vi "process_storage.vi"() -> ()   [LabVIEW 2011, in "Fiberscope_library.lvlib"]
uses:
  Fiberscope_library.lvlib
  typedefs/element_images_cluster.ctl
  typedefs/control_process_state_cluster.ctl
  typedefs/control_process_state_enum.ctl
  typedefs/feedback_to_watchdog.ctl
  typedefs/feedback_from_process_enum.ctl
  typedefs/all_scan_parameters_cluster.ctl
  typedefs/fiber_parameters_cluster.ctl
  typedefs/spiral_parameters_cluster.ctl
  typedefs/run_parameters_cluster.ctl
  typedefs/run_mode_enum.ctl
  typedefs/acquisition_parameters_cluster.ctl
  typedefs/image_size_I32.ctl
  typedefs/smooth_coeffs_cluster.ctl
  typedefs/storage_parameters_cluster.ctl
panel:
  out "Local exit":bool
  out "Last saved image":string
  out "error out":errorcluster
  in  "error in":errorcluster
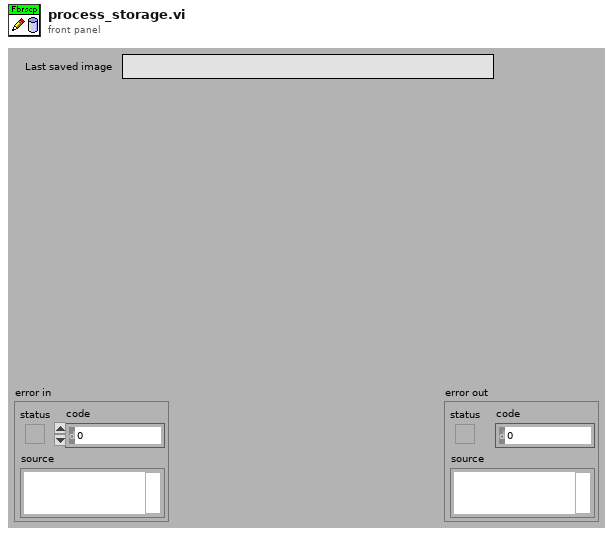
[diagram p1: front panel]
types:
  T1 = typedef "Fiberscope_library.lvlib/feedback_to_watchdog.ctl" = cluster{"Feedback_from_process_enum":T2, "Process_name":string}
  T2 = typedef "Fiberscope_library.lvlib/feedback_from_process_enum.ctl" = enum16{"Has_initialised", "Changed_parameters", "Has_started", "Has_stopped", "Has_quitted", "Is_running", "Has_finished", "Custom"}
  T3 = typedef "Fiberscope_library.lvlib/control_process_state_cluster.ctl" = cluster{"Control_process_state_enum":T4, "variant":variant}
  T4 = typedef "Fiberscope_library.lvlib/control_process_state_enum.ctl" = enum16{"Init", "Quit", "Start", "Stop", "Change_parameters", "Running", "Finish", "Custom"}
  T5 = typedef "Fiberscope_library.lvlib/element_images_cluster.ctl" = cluster{"Images_array":dbl[][][], "#channels":i32, "Last element?":bool}
  T6 = typedef "Fiberscope_library.lvlib/all_scan_parameters_cluster.ctl" = cluster{"Fiber parameters":T7, "Spiral parameters":T8, "Run parameters":T9, "Acquisition parameters":T11, "Fiber parameters pixel_mapper":T7, "Smooth_coeffs_cluster":T13, "Storage parameters":T14}
  T7 = typedef "Fiberscope_library.lvlib/fiber_parameters_cluster.ctl" = cluster{"Frequency":dbl, "Amplitude X":dbl, "Amplitude Y":dbl, "Initial Amplitude X":dbl, "Initial Amplitude Y":dbl, "Phase":dbl}
  T8 = typedef "Fiberscope_library.lvlib/spiral_parameters_cluster.ctl" = cluster{"Imaging periods":dbl, "Settling periods":dbl, "Resting periods":dbl}
  T9 = typedef "Fiberscope_library.lvlib/run_parameters_cluster.ctl" = cluster{"Run mode":T10, "Averages per frame":u8, "No. of frames":u32}
  T10 = typedef "Fiberscope_library.lvlib/run_mode_enum.ctl" = enum16{"Continuous", "Single frame", "No. of frames"}
  T11 = typedef "Fiberscope_library.lvlib/acquisition_parameters_cluster.ctl" = cluster{"Cycles per pixel":u32, "Image size":T12}
  T12 = typedef "Fiberscope_library.lvlib/image_size_I32.ctl" = i32
  T13 = typedef "Fiberscope_library.lvlib/smooth_coeffs_cluster.ctl" = cluster{"Coeff 1":dbl, "Coeff 2":dbl}
  T14 = typedef "Fiberscope_library.lvlib/storage_parameters_cluster.ctl" = cluster{"Autosave":bool, "Path":path}
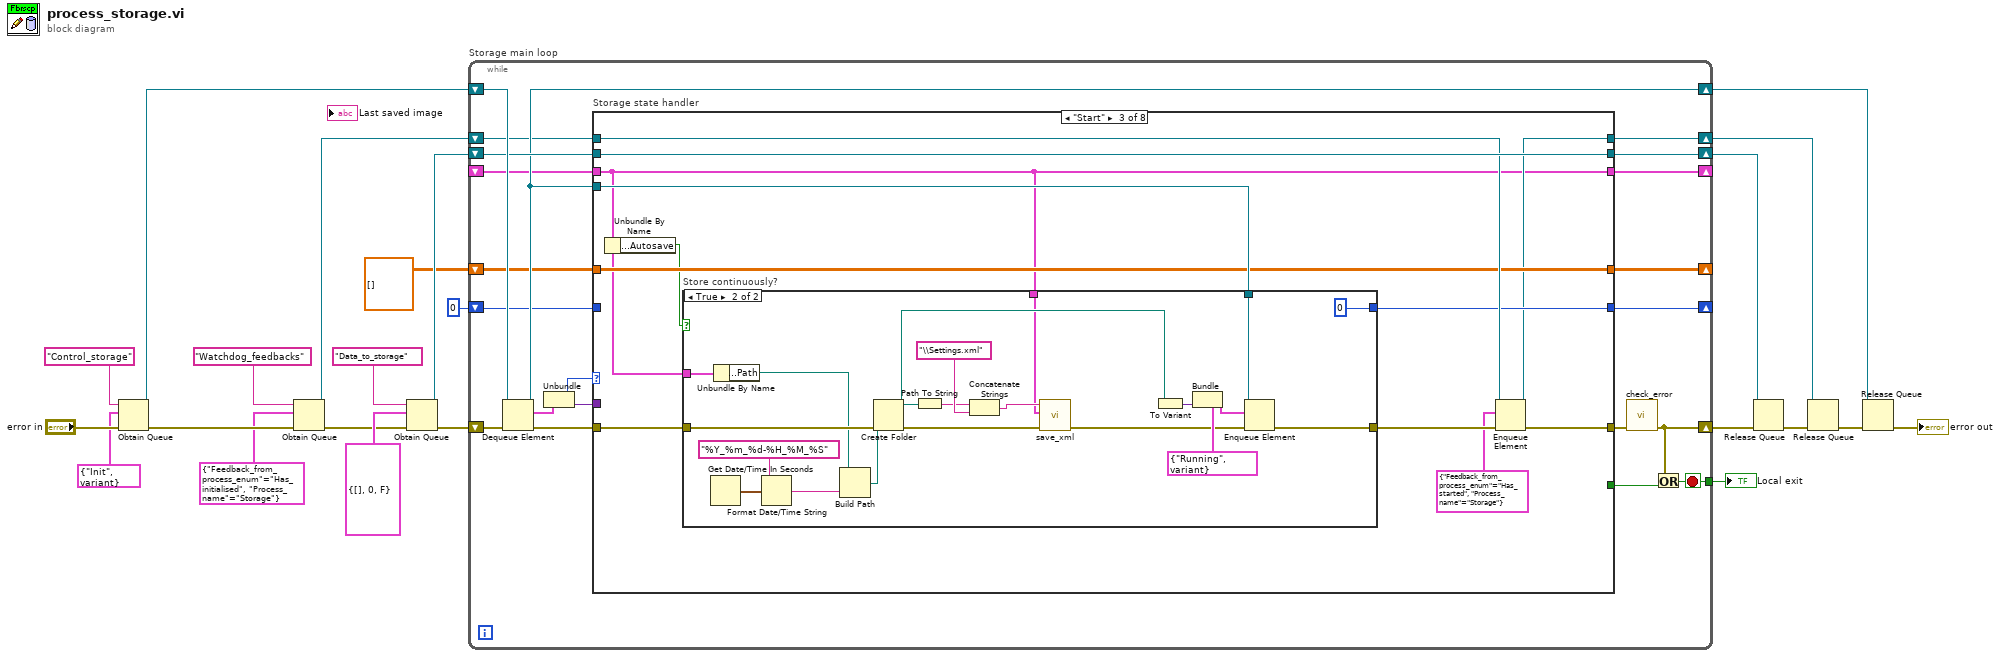
[diagram p0: block diagram]
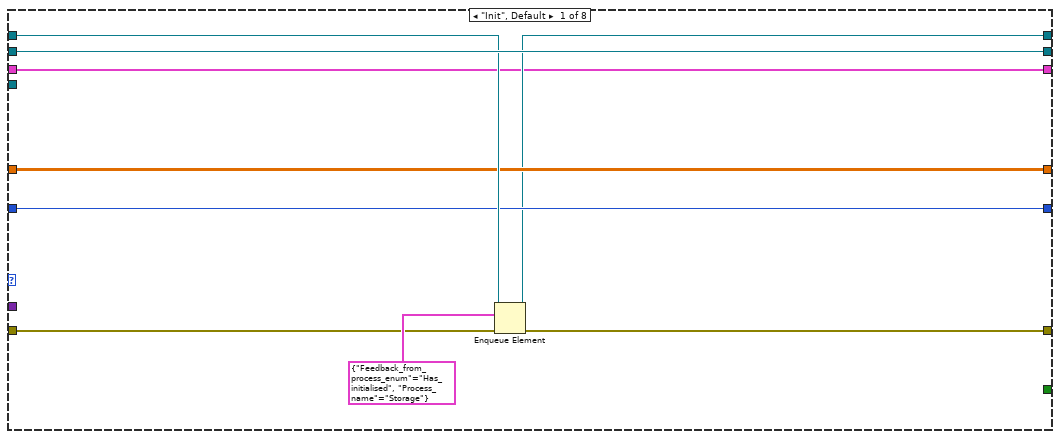
[diagram p2: hidden frame]
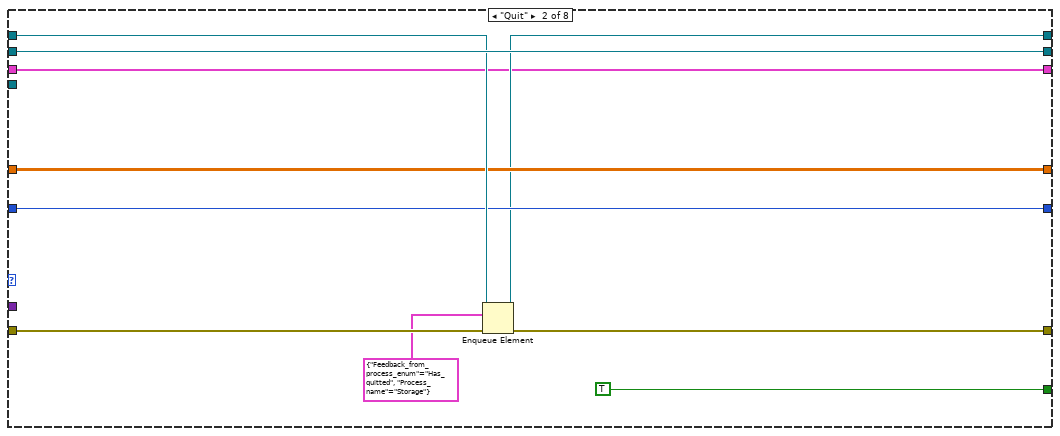
[diagram p3: hidden frame]
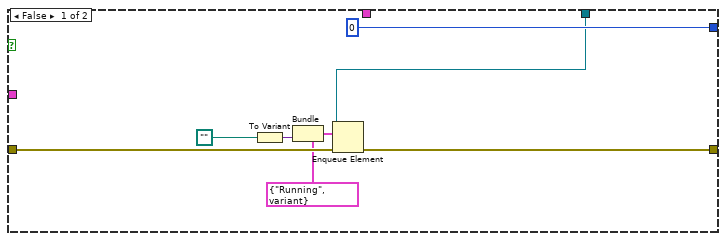
[diagram p4: hidden frame]
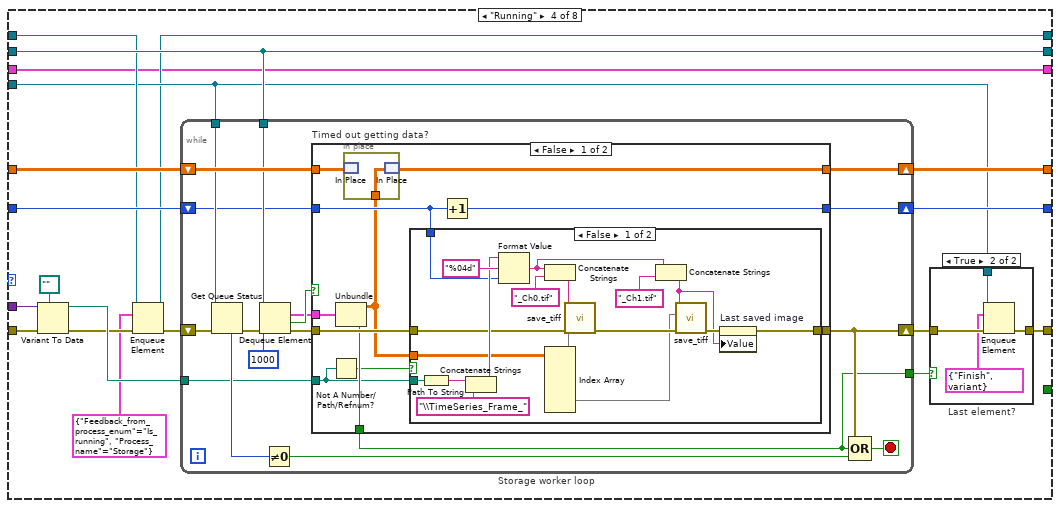
[diagram p5: hidden frame]
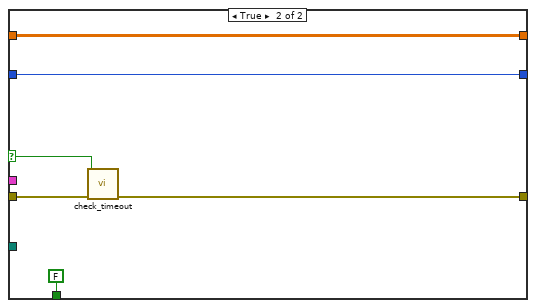
[diagram p8: hidden frame]
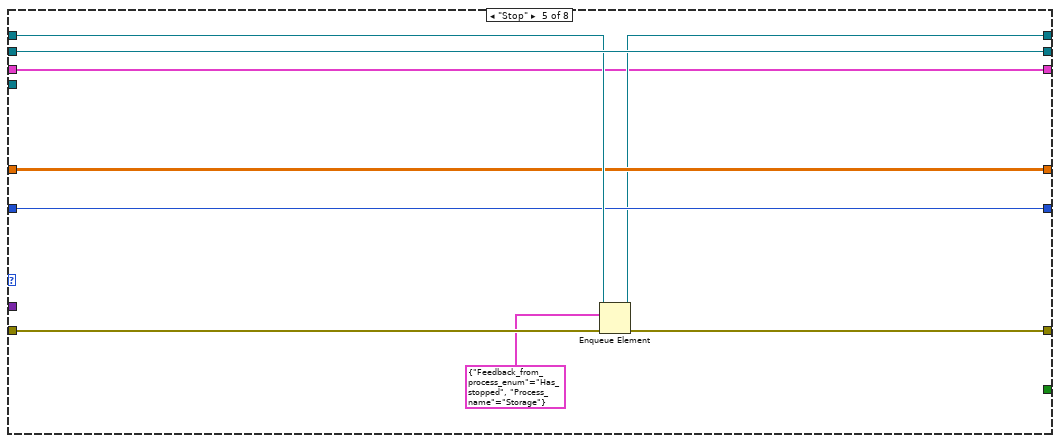
[diagram p9: hidden frame]
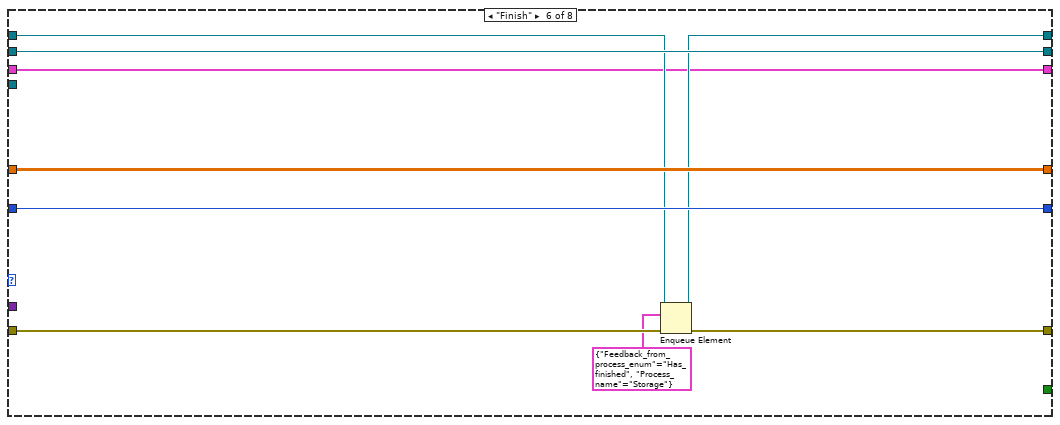
[diagram p10: hidden frame]
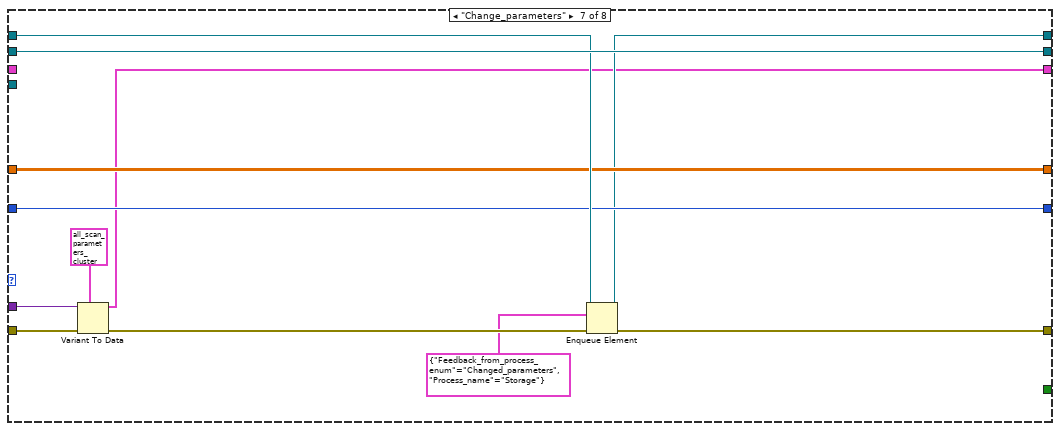
[diagram p11: hidden frame]
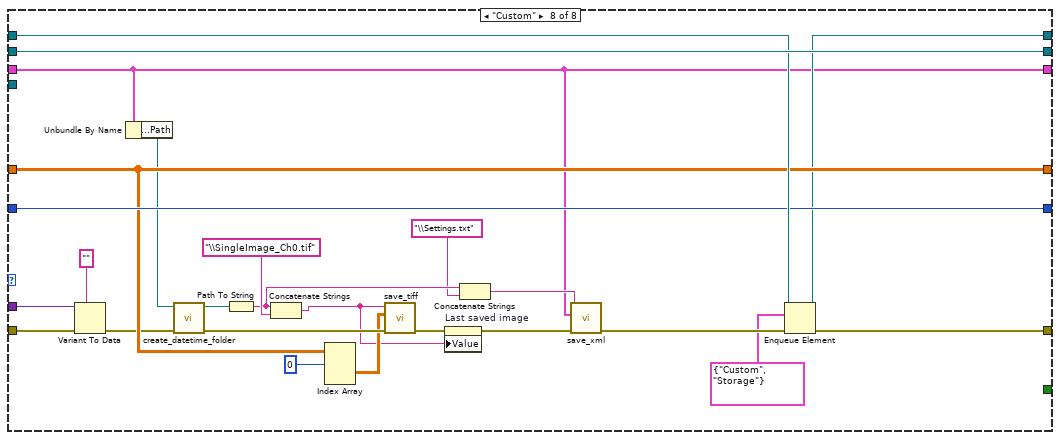
[diagram p12: hidden frame]
diagram:
  n1 = Obtain Queue(name (unnamed)="Control_storage", element data type=T3 {"Control_process_state_enum"=enum."Init", "variant"=variant} ("Control_process_state_cluster"), error in (no error)="error in") -> (queue out=w7:refnum<queue>, error out=w6:errorcluster)  [unwired: 2 in, 1 out]
  n2 = Obtain Queue(name (unnamed)="Watchdog_feedbacks", element data type=T1 {"Feedback_from_process_enum"=enum."Has_initialised", "Process_name"="Storage"}, error in (no error)=w6) -> (queue out=w12:refnum<queue>, error out=w14:errorcluster)  [unwired: 2 in, 1 out]
  n3 = Obtain Queue(name (unnamed)="Data_to_storage", element data type=T5 {"Images_array"=[], "#channels"=0, "Last element?"=FALSE}, error in (no error)=w14) -> (queue out=w19:refnum<queue>, error out=w20:errorcluster)  [unwired: 2 in, 1 out]
  n4 = while "Storage main loop" {
    shift-right: [w27] -> w17
    shift-left: w20 -> [w44]
    shift-right: [w35] -> w15
    shift-left: w7 -> [w43]
    shift-right: [w37] -> w16
    shift-left: w19 -> [w38]
    shift-right: [w26] -> w9
    shift-left: w12 -> [w33]
    shift-right: [w32] -> _
    shift-left: dbl[][][] [] ("Images_array") -> [w31]
    tunnel: [w30] -> w8
    shift-right: [w29] -> _
    shift-left: 0 -> [w28]
    shift-right: [w25] -> _
    shift-left: _ -> [w24]
    stop <- w30 stop-if-true
    n5 = Dequeue Element(queue=w43, error in (no error)=w44) -> (queue out=w35:refnum<queue>, element=w41:T3, error out=w42:errorcluster)  [unwired: 1 in, 1 out]
    n6 = Unbundle(w41) -> ("Control_process_state_enum"=w40:T4, "variant"=w34:variant)
    n7 = case "Storage state handler" shown="\"Start\"" w40 {
      tunnel: w42 -> [w45 w61 w72 w120 w190 w197 w211 w225]
      tunnel: [w52 w60 w68 w109 w189 w196 w208 w236] -> w36
      tunnel: [_ TRUE _ _ _ _ _ _] -> w39
      tunnel: w38 -> [w53 w62 w75 w115 w191 w200 w212 w237]
      tunnel: [w53 w62 w75 w115 w191 w200 w212 w237] -> w37
      tunnel: w35 -> [_ _ w73 w108 _ _ _ _]
      tunnel: w34 -> [_ _ _ w119 _ _ w210 w223]
      tunnel: w33 -> [w51 w59 w74 w111 w188 w195 w207 w235]
      tunnel: [w50 w58 w71 w122 w187 w199 w206 w228] -> w32
      tunnel: w31 -> [w50 w58 w71 w121 w187 w199 w206 w228]
      tunnel: [w49 w57 w70 w116 w186 w198 w205 w230] -> w29
      tunnel: w28 -> [w49 w57 _ w117 w186 w198 w205 w230]
      tunnel: [w48 w56 w67 w106 w185 w194 w204 w217] -> w26
      tunnel: [w46 w54 w64 w104 w183 w192 w202 w213] -> w25
      tunnel: w24 -> [w46 w54 w64 w104 w183 w192 _ w213]
      frame "Init", Default {
        n8 = Enqueue Element(queue=w51, element=T1 {"Feedback_from_process_enum"=enum."Has_initialised", "Process_name"="Storage"}, error in (no error)=w45) -> (queue out=w48:refnum<queue>, error out=w52:errorcluster)  [unwired: 1 in, 1 out]
      }
      frame "Quit" {
        n9 = Enqueue Element(queue=w59, element=T1 {"Feedback_from_process_enum"=enum."Has_quitted", "Process_name"="Storage"}, error in (no error)=w61) -> (queue out=w56:refnum<queue>, error out=w60:errorcluster)  [unwired: 1 in, 1 out]
      }
      frame "Start" {
        n10 = Unbundle By Name(w64) -> ("Storage parameters.Autosave"=w65:bool)
        n11 = case "Store continuously?" shown="True" w65 {
          tunnel: w73 -> [w80 w103]
          tunnel: w72 -> [w82 w98]
          tunnel: [0 0] -> w70
          tunnel: [w81 w96] -> w69
          tunnel: w64 -> [_ w84]
          tunnel: w64 -> [_ w86]
          frame False {
            n12 = To Variant(anything=path "") -> (Variant=w77:variant)
            n13 = Bundle(cluster=T3 {"Control_process_state_enum"=enum."Running", "variant"=variant} ("Control_process_state_cluster"), "variant"=w77) -> (w78:T3)  [unwired: 1 in]
            n14 = Enqueue Element(queue=w80, element=w78, error in (no error)=w82) -> (error out=w81:errorcluster)  [unwired: 1 in, 2 out]
          }
          frame True {
            n15 = Get Date/Time In Seconds() -> (seconds since 1Jan1904=w102:timestamp)
            n16 = Unbundle By Name(w86) -> ("Storage parameters.Path"=w85:path)
            n17 = Format Date/Time String(time format string (%c)="%Y_%m_%d-%H_%M_%S", seconds (now)=w102) -> (date/time string=w101:string)  [unwired: 1 in]
            n18 = Build Path(base path=w85, name or relative path=w101) -> (appended path=w99:path)
            n19 = Create Folder(path (use dialog)=w99, error in=w98) -> (created path=w91:path, error out=w88:errorcluster)  [unwired: 1 in, 1 out]
            n20 = Path To String(path=w91) -> (string=w90:string)
            n21 = Concatenate Strings(w90, "\\Settings.xml" ("string")) -> (w89:string)
            n22 = call "save_xml.vi"("error in"=w88, "All scan parameters"=w84, "Path"=w89) -> ("error out"=w87:errorcluster)  [unwired: 8 in]
            n23 = To Variant(anything=w91) -> (Variant=w95:variant)
            n24 = Bundle(cluster=T3 {"Control_process_state_enum"=enum."Running", "variant"=variant} ("Control_process_state_cluster"), "variant"=w95) -> (w94:T3)  [unwired: 1 in]
            n25 = Enqueue Element(queue=w103, element=w94, error in (no error)=w87) -> (error out=w96:errorcluster)  [unwired: 1 in, 2 out]
          }
        }
        n26 = Enqueue Element(queue=w74, element=T1 {"Feedback_from_process_enum"=enum."Has_started", "Process_name"="Storage"}, error in (no error)=w69) -> (queue out=w67:refnum<queue>, error out=w68:errorcluster)  [unwired: 1 in, 1 out]
      }
      frame "Running" {
        n27 = Variant To Data(error in=w120, type=path "" ("Path"), Variant=w119) -> (data=w114:path, error out=w113:errorcluster)
        n28 = Enqueue Element(queue=w111, element=T1 {"Feedback_from_process_enum"=enum."Is_running", "Process_name"="Storage"}, error in (no error)=w113) -> (queue out=w106:refnum<queue>, error out=w112:errorcluster)  [unwired: 1 in, 1 out]
        n29 = while "Storage worker loop" {
          shift-right: [w129] -> w110
          shift-left: w112 -> [w145]
          shift-right: [w136] -> w122
          shift-left: w121 -> [w135]
          shift-right: [w130] -> w116
          shift-left: w117 -> [w131]
          tunnel: w108 -> [w134]
          tunnel: w115 -> [w133]
          tunnel: w114 -> [w132]
          tunnel: [w128] -> w107
          stop <- w142 stop-if-true
          n30 = Get Queue Status(queue=w134, error in (no error)=w145) -> (error out=w144:errorcluster, # elements in queue=w143:i32)  [unwired: 1 in, 6 out]
          n31 = Dequeue Element(queue=w133, timeout in ms (-1)=1000, error in (no error)=w144) -> (element=w137:T5, timed out?=w138:bool, error out=w139:errorcluster)  [unwired: 1 out]
          n32 = Not Equal To 0?(x=w143) -> (x != 0?=w141:bool)
          n33 = case "Timed out getting data?" shown="False" w138 {
            selector: w138 -> [_ w180]
            tunnel: w139 -> [w154 w182]
            tunnel: [w153 w181] -> w129
            tunnel: w137 -> [w152 _]
            tunnel: [w146 w179] -> w136
            tunnel: w135 -> [w148 w179]
            tunnel: w132 -> [w150 _]
            tunnel: w131 -> [w156 w178]
            tunnel: [w155 w178] -> w130
            tunnel: [w151 FALSE ("Last element?")] -> w128
            frame False {
              n34 = Not A Number/Path/Refnum?(number/path/refnum=w150) -> (NaN/Path/Refnum?=w149:bool)
              n35 = Unbundle(w152) -> ("Images_array"=w147:dbl[][][], "Last element?"=w151:bool)  [unwired: 1 out]
              n36 = in-place {
                in-place-border: w147 -> [w157]
                n37 = in-place-match #1(w148) -> ()  [unwired: 1 out]
                n38 = in-place-match #1(w157) -> (w146:dbl[][][])
              }
              n39 = case shown="False" w149 {
                tunnel: w150 -> [w173 _]
                tunnel: w156 -> [w169 _]
                tunnel: w154 -> [w168 w176]
                tunnel: [w166 w176] -> w153
                tunnel: w147 -> [w164 _]
                frame False {
                  n40 = Path To String(path=w173) -> (string=w175:string)
                  n41 = Concatenate Strings(w175, "\\TimeSeries_Frame_" ("string")) -> (w171:string)
                  n42 = Format Value(string ("")=w171, format string="%04d", value (0)=w169) -> (output string=w161:string)
                  n43 = Concatenate Strings(w161, "_Ch0.tif" ("string")) -> (w165:string)
                  n44 = Index Array(array=w164) -> (element #1=w167:dbl[][], element #2=w159:dbl[][])  [unwired: 6 in]
                  n45 = call "save_tiff.vi"("error in (no error)"=w168, "Data"=w167, "Path"=w165) -> ("error out"=w163:errorcluster)  [unwired: 8 in]
                  n46 = Concatenate Strings(w161, "_Ch1.tif" ("string")) -> (w158:string)
                  n47 = call "save_tiff.vi"("error in (no error)"=w163, "Data"=w159, "Path"=w158) -> ("error out"=w162:errorcluster)  [unwired: 8 in]
                  n48 = property on="Last saved image" class="Str"(error in=w162, "Value"=w158) -> (error out=w166:errorcluster)  [unwired: 1 in, 1 out]
                }
                frame True {
                  # "No valid path provided\n-> do not store continuously!"
                }
              }
              n49 = Increment(x=w156) -> (x+1=w155:i32)
            }
            frame True {
              n50 = call "check_timeout.vi"("error in"=w182, "Timeout?"=w180) -> ("error out"=w181:errorcluster)  [unwired: 9 in]
            }
          }
          n51 = Compound Arithmetic op=OR(w129, w128, w141) -> (w142:bool)
        }
        n52 = case "Last element?" shown="True" w107 {
          tunnel: w110 -> [w123 w127]
          tunnel: [w123 w126] -> w109
          tunnel: w108 -> [_ w125]
          frame False {
          }
          frame True {
            n53 = Enqueue Element(queue=w125, element=T3 {"Control_process_state_enum"=enum."Finish", "variant"=variant} ("Control_process_state_cluster"), error in (no error)=w127) -> (error out=w126:errorcluster)  [unwired: 1 in, 2 out]
          }
        }
      }
      frame "Stop" {
        n54 = Enqueue Element(queue=w188, element=T1 {"Feedback_from_process_enum"=enum."Has_stopped", "Process_name"="Storage"}, error in (no error)=w190) -> (queue out=w185:refnum<queue>, error out=w189:errorcluster)  [unwired: 1 in, 1 out]
      }
      frame "Finish" {
        n55 = Enqueue Element(queue=w195, element=T1 {"Feedback_from_process_enum"=enum."Has_finished", "Process_name"="Storage"}, error in (no error)=w197) -> (queue out=w194:refnum<queue>, error out=w196:errorcluster)  [unwired: 1 in, 1 out]
      }
      frame "Change_parameters" {
        n56 = Variant To Data(error in=w211, type=T6 {"Fiber parameters"={"Frequency"=100.0, "Amplitude X"=0.0, "Amplitude Y"=0.0, "Initial Amplitude X"=0.0, "Initial Amplitude Y"=0.0, "Phase"=0.0}, "Spiral parameters"={"Imaging periods"=1.0, "Settling periods"=1.0, "Resting periods"=1.0}, "Run parameters"={"Run mode"=enum."Continuous", "Averages per frame"=1, "No. of frames"=1}, "Acquisition parameters"={"Cycles per pixel"=1, "Image size"=128}, "Fiber parameters pixel_mapper"={"Frequency"=100.0, "Amplitude X"=0.0, "Amplitude Y"=0.0, "Initial Amplitude X"=0.0, "Initial Amplitude Y"=0.0, "Phase"=0.0}, "Smooth_coeffs_cluster"={"Coeff 1"=0.0, "Coeff 2"=0.0}, "Storage parameters"={"Autosave"=FALSE, "Path"=path "D:/"}} ("All scan parameters"), Variant=w210) -> (data=w202:T6, error out=w209:errorcluster)
        n57 = Enqueue Element(queue=w207, element=T1 {"Feedback_from_process_enum"=enum."Changed_parameters", "Process_name"="Storage"}, error in (no error)=w209) -> (queue out=w204:refnum<queue>, error out=w208:errorcluster)  [unwired: 1 in, 1 out]
      }
      frame "Custom" {
        n58 = Variant To Data(error in=w225, type="" ("Comment"), Variant=w223) -> (error out=w224:errorcluster)  [unwired: 1 out]
        n59 = Unbundle By Name(w213) -> ("Storage parameters.Path"=w214:path)
        n60 = call "create_datetime_folder.vi"("error in (no error)"=w224, "Path"=w214) -> ("error out"=w232:errorcluster, "created path"=w233:path)  [unwired: 8 in]
        n61 = Path To String(path=w233) -> (string=w222:string)
        n62 = Concatenate Strings(w222, "\\SingleImage_Ch0.tif" ("string")) -> (w226:string)
        n63 = Index Array(array=w228, index (dim 0)=0 ("disabled index (row)")) -> (element=w229:dbl[][])  [unwired: 2 in]
        n64 = call "save_tiff.vi"("error in (no error)"=w232, "Data"=w229, "Path"=w226) -> ("error out"=w227:errorcluster)  [unwired: 8 in]
        n65 = property on="Last saved image" class="Str"(error in=w227, "Value"=w226) -> (error out=w220:errorcluster)  [unwired: 1 in, 1 out]
        n66 = Concatenate Strings(w222, "\\Settings.txt" ("string")) -> (w218:string)
        n67 = call "save_xml.vi"("error in"=w220, "All scan parameters"=w213, "Path"=w218) -> ("error out"=w219:errorcluster)  [unwired: 8 in]
        n68 = Enqueue Element(queue=w235, element=T1 {"Feedback_from_process_enum"=enum."Custom", "Process_name"="Storage"}, error in (no error)=w219) -> (queue out=w217:refnum<queue>, error out=w236:errorcluster)  [unwired: 1 in, 1 out]
      }
    }
    n69 = call "check_error.vi"("error in"=w36) -> ("error out"=w27:errorcluster)  [unwired: 10 in]
    n70 = Or(x=w27, y=w39) -> (x .or. y?=w30:bool)
  }
  "Local exit" <- w8
  n71 = Release Queue(queue=w16, error in (no error)=w17) -> (error out=w11:errorcluster)  [unwired: 1 in, 2 out]
  n72 = Release Queue(queue=w9, error in (no error)=w11) -> (error out=w10:errorcluster)  [unwired: 1 in, 2 out]
  n73 = Release Queue(queue=w15, error in (no error)=w10) -> (error out=→"error out":errorcluster)  [unwired: 1 in, 2 out]
